vi "Timer_ext.vi"(4 "tick old":u32, 6 "t ms old":u32, 8 "ms":u32, 9 "Load":bool, 10 "Reset":bool, 11 "Start":bool) -> (1 "tick":u32, 2 "t ms":u32, 3 "End":bool)   [LabVIEW 2019, in "Timers.lvlib"]
uses:
  Timers.lvlib
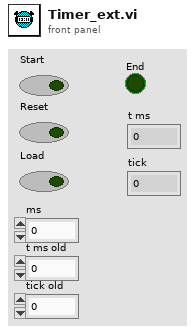
[diagram p1: front panel]
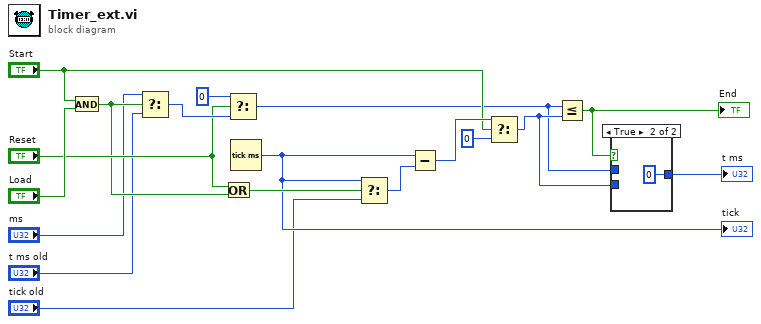
[diagram p0: block diagram]
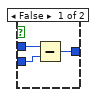
[diagram p2: hidden frame]
diagram:
  n1 = And(x="Start", y="Load") -> (x .and. y?=w13:bool)
  n2 = Select(t="ms", s=w13, f="t ms old") -> (s? t:f=w16:u32)
  n3 = Or(x="Reset", y=w13) -> (x .or. y?=w18:bool)
  n4 = Select(t=u32 0, s="Reset", f=w16) -> (s? t:f=w5:u32)
  n5 = Tick Count (ms)() -> (millisecond timer value=w2:u32)
  "tick" <- w2
  n6 = Select(t=w2, s=w18, f="tick old") -> (s? t:f=w4:u32)
  n7 = Subtract(x=w2, y=w4) -> (x-y=w10:u32)
  n8 = Select(t=w10, s="Start", f=u32 0) -> (s? t:f=w6:u32)
  n9 = Less Or Equal?(x=w5, y=w6) -> (x <= y?=w12:bool)
  "End" <- w12
  n10 = case shown="True" w12 {
    tunnel: w6 -> [w20 _]
    tunnel: [w21 u32 0] -> w11
    tunnel: w5 -> [w19 _]
    frame False {
      n11 = Subtract(x=w19, y=w20) -> (x-y=w21:u32)
    }
    frame True {
    }
  }
  "t ms" <- w11
